vi "Write ServerName.vi"(8 "error in (no error)":errorcluster, 10 "ServerName":string, 11 "DIMActor in":refnum<class "DIMActor.lvclass">) -> (0 "error out":errorcluster, 3 "DIMActor out":refnum<class "DIMActor.lvclass">)   [LabVIEW 2012, in "DIMActor.lvlib" / "DIMActor.lvclass"]
doc: "Set DIM server name."
uses:
  DIMActor.lvclass
  DIMActor.lvclass/DIMActor.ctl
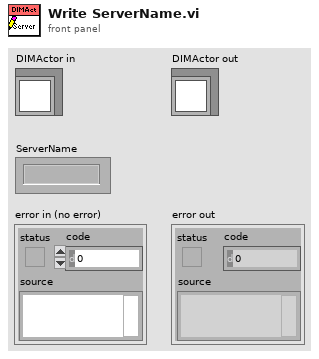
[diagram p1: front panel]
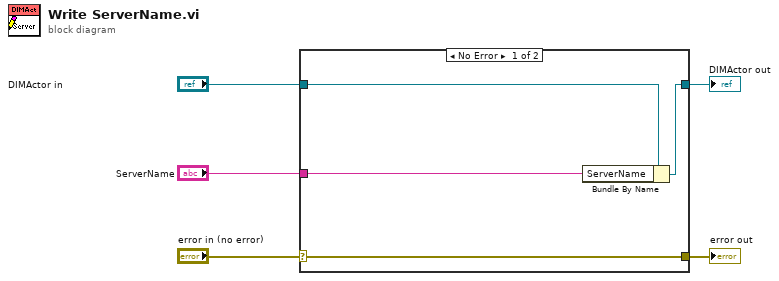
[diagram p0: block diagram]
diagram:
  n1 = case shown="No Error" "error in (no error)" {
    selector: "error in (no error)" -> [w9 w10]
    tunnel: [w9 w10] -> w4
    tunnel: [w7 w11] -> w2
    tunnel: "DIMActor in" -> [w8 w11]
    tunnel: "ServerName" -> [w6 _]
    frame No Error {
      n2 = Bundle By Name(cluster=w8, "ServerName"=w6) -> (w7:refnum<class "DIMActor.lvclass">)
    }
    frame Error {
    }
  }
  "error out" <- w4
  "DIMActor out" <- w2
